vi "Mic_Grab.vi"(6 "Input":u16(ring) items=["Hammer (force)", "Self-tap", "Spacebar"], 7 "Ports":cluster{"mic":u8, "hammer":u8, "flip?":bool}={"mic"=1, "hammer"=2, "flip?"=FALSE}, 8 "error In":errorcluster, 9 "Threshold":dbl, 10 "Pre-trigger (s)":dbl=0.01 format="%#_13g", 11 "DAQ Prams":T4={"task ID"=0, "Num Pts"=0, "timeout"=0.0, "FIFO"=0, "Double Bounce"=1.0} {"Double Bounce" format="%#.2g"; "task ID" format="%.0x"}) -> (0 "error out":errorcluster, 1 "latest data":waveform(dbl)[](array[waveform]), 2 "Full":bool, 3 "DAQ Prams":T4={"task ID"=0, "Num Pts"=0, "timeout"=0.0, "FIFO"=0, "Double Bounce"=1.0} {"Double Bounce" format="%#.2g"; "task ID" format="%.0x"}, 4 "Start Task":T2(ring), 5 "Tap":T1)   [LabVIEW 2022 SP3]
uses:
  <vilib>/sound2/lvsound2.llb/Sound Input Task ID.ctl
  <extravilib>/ChannelInstances/Lossy Stream-a[.](wfm(dbl))/)Channel.ctl
  <extravilib>/ChannelInstances/Lossy Stream-a[.](wfm(dbl))/Write With Abort.vi
  <extravilib>/ChannelInstances/Lossy Stream-a[.](wfm(dbl))/Endpoint.vi
  Mic_Global.vi
  <vilib>/sound2/lvsound2.llb/Sound Input Read (DBL).vi
  <extravilib>/ChannelInstances/Lossy Stream-a[.](wfm(dbl))/)Channel.vi
  <extravilib>/ChannelInstances/Lossy Stream-a[.](wfm(dbl)).lvlib
panel:
  # "microphone, hammer"
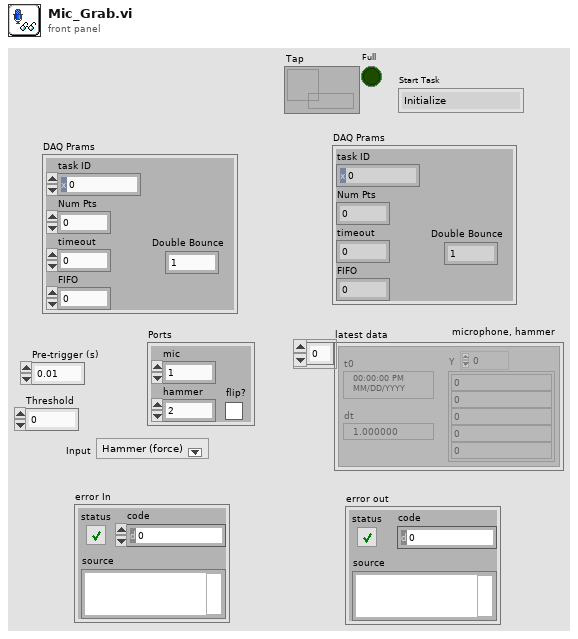
[diagram p1: front panel]
types:
  T1 = typedef "Lossy Stream-a[.](wfm(dbl)).lvlib/)Channel.ctl" = refnum<queue>
  T2 = enum16{"Initialize", "Free run", "One Shot - waiting", "One Shot - triggered", "Wait", "Close"}
  T3 = typedef "Sound Input Task ID.ctl" = u32
  T4 = cluster{"task ID":T3, "Num Pts":i32, "timeout":dbl, "FIFO":i32, "Double Bounce":dbl}
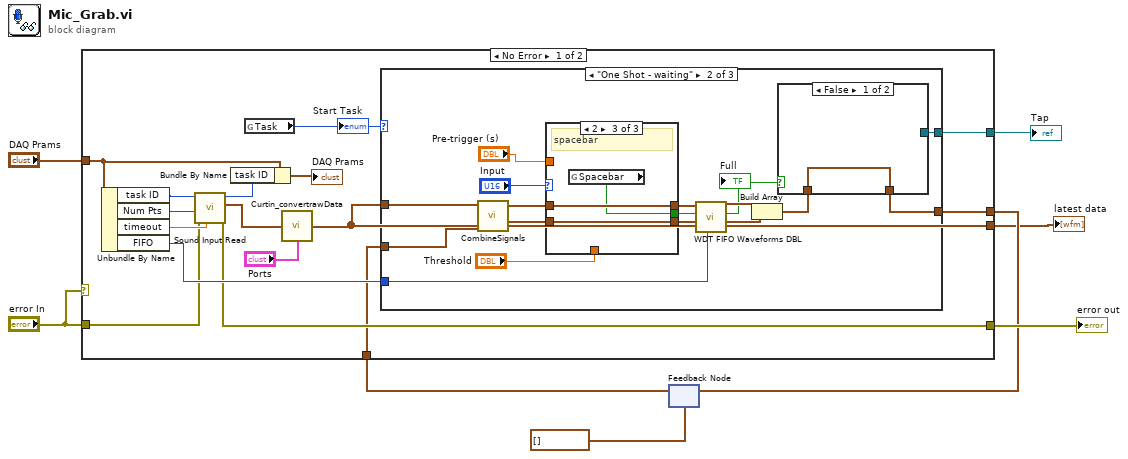
[diagram p0: block diagram]
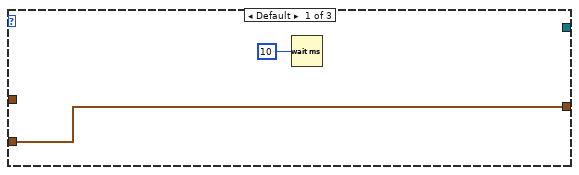
[diagram p2: hidden frame]
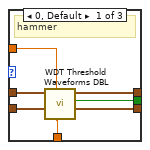
[diagram p3: hidden frame]
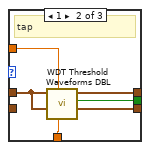
[diagram p4: hidden frame]
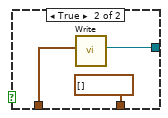
[diagram p5: hidden frame]
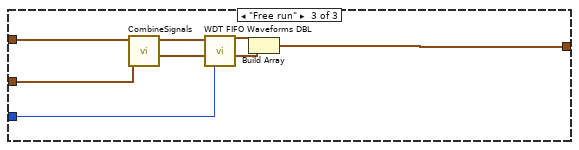
[diagram p6: hidden frame]
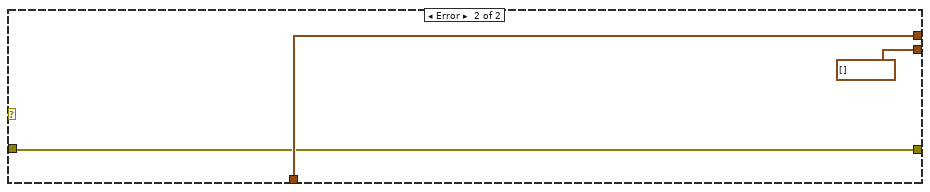
[diagram p7: hidden frame]
diagram:
  n1 = feedback #1(waveform(dbl)[] []) -> (w5:waveform(dbl)[])
  n2 = case shown="No Error" "error In" {
    tunnel: "DAQ Prams" -> [w19 _]
    tunnel: "error In" -> [w16 w73]
    tunnel: [w15 w73] -> w7
    tunnel: [w14 w74] -> w6
    tunnel: w5 -> [w13 w74]
    tunnel: [w10 _] -> w2
    tunnel: [w9 waveform(dbl)[] []] -> w1
    frame No Error {
      n3 = Unbundle By Name(w19) -> ("task ID"=w23:T3, "Num Pts"=w22:i32, "timeout"=w21:dbl, "FIFO"=w17:i32)
      n4 = call-poly <vilib>:"Sound Input Read.vi"("timeout (sec)"=w21, "number of samples/ch"=w22, "error in (no error)"=w16, "task ID"=w23) -> ("error out"=w15:errorcluster, "data"=w24:waveform(dbl)[], "task ID out"=w20:T3)  [unwired: 5 in]
      n5 = Bundle By Name(cluster=w19, "task ID"=w20) -> (→"DAQ Prams":T4)
      n6 = global read "Mic_Global.vi" "Task"() -> (w12:T2)
      "Start Task" <- w12
      n7 = call "Curtin_convertrawData.vi"("incoming data"=w24, "Ports"="Ports") -> ("Ordered"=w9:waveform(dbl)[])
      n8 = case shown="\"One Shot - waiting\"" w12 {
        tunnel: w9 -> [_ w35 w71]
        tunnel: w13 -> [w26 w34 w66]
        tunnel: [w26 w37 w67] -> w14
        tunnel: w17 -> [_ w41 w68]
        tunnel: [_ w38 _] -> w10
        frame Default {
          n9 = Wait (ms)(milliseconds to wait=u32 10) -> ()  [unwired: 1 out]
        }
        frame "One Shot - waiting" {
          n10 = call "CombineSignals.vi"("Old signal"=w34, "New signal"=w35) -> ("Ch 2"=w32:waveform(dbl), "Ch 1"=w33:waveform(dbl))  [unwired: 8 in]
          n11 = case shown="2" "Input" {
            tunnel: w32 -> [w49 _ w58]
            tunnel: w33 -> [w48 w56 w59]
            tunnel: "Threshold" -> [w50 w52 _]
            tunnel: "Pre-trigger (s)" -> [w44 w51 _]
            tunnel: [w47 w53 w58] -> w29
            tunnel: [w46 w54 w57] -> w28
            tunnel: [w45 w55 w59] -> w27
            frame 0, Default {
              # "hammer"
              n12 = call "WDT Threshold Waveforms DBL.vi"("A Threshold"=w50, "Pre-trigger (s)"=w44, "Hammer"=w49, "Mic"=w48) -> ("Hammer out"=w47:waveform(dbl), "Triggered?"=w46:bool, "Mic out"=w45:waveform(dbl))  [unwired: 4 in, 1 out]
            }
            frame 1 {
              # "tap"
              n13 = call "WDT Threshold Waveforms DBL.vi"("A Threshold"=w52, "Pre-trigger (s)"=w51, "Hammer"=w56, "Mic"=w56) -> ("Hammer out"=w53:waveform(dbl), "Triggered?"=w54:bool, "Mic out"=w55:waveform(dbl))  [unwired: 4 in, 1 out]
            }
            frame 2 {
              # "spacebar"
              n14 = global read "Mic_Global.vi" "Spacebar"() -> (w57:bool)
            }
          }
          n15 = call "WDT FIFO Waveforms DBL.vi"("FIFO"=w41, "Hammer"=w29, "Triggered?"=w28, "Mic"=w27) -> ("Hammer out"=w43:waveform(dbl), "Full"=w40:bool, "Mic out"=w42:waveform(dbl))  [unwired: 4 in, 1 out]
          "Full" <- w40
          n16 = Build Array(w42, w43) -> (w39:waveform(dbl)[])
          n17 = case shown="False" w40 {
            tunnel: w39 -> [w60 w63]
            tunnel: [_ w62] -> w38
            tunnel: [w60 waveform(dbl)[] []] -> w37
            frame False {
            }
            frame True {
              n18 = call <extravilib>:"Write.vi"("element"=w63) -> ("channel"=w62:T1)  [unwired: 8 in, 2 out]
            }
          }
        }
        frame "Free run" {
          n19 = call "CombineSignals.vi"("Old signal"=w66, "New signal"=w71) -> ("Ch 2"=w64:waveform(dbl), "Ch 1"=w65:waveform(dbl))  [unwired: 8 in]
          n20 = call "WDT FIFO Waveforms DBL.vi"("FIFO"=w68, "Hammer"=w64, "Mic"=w65) -> ("Hammer out"=w70:waveform(dbl), "Mic out"=w69:waveform(dbl))  [unwired: 5 in, 2 out]
          n21 = Build Array(w69, w70) -> (w67:waveform(dbl)[])
        }
      }
    }
    frame Error {
    }
  }
  "latest data" <- w1
  "error out" <- w7
  "Tap" <- w2
  n22 = feedback-in #1(w6) -> ()
